vi "Generate Simulated Channel Block.vi"(8 "error in (no error)":errorcluster, 9 "Target Size (bytes)":i32, 10 "Number of Channels":i32, 11 "Simulated VeriStand Engine in":refnum<class "Simulated VeriStand Engine.lvclass">) -> (0 "error out":errorcluster, 1 "Actual Size (bytes)":i32, 2 "Channels":T1[](array[typedef]), 3 "Simulated VeriStand Engine out":refnum<class "Simulated VeriStand Engine.lvclass">)   [LabVIEW 2016, in "Simulated VeriStand Engine.lvclass"]
uses:
  Simulated VeriStand Engine.lvclass
  <vilib>/NI Veristand/VeriStand Data/Typedefs/Typedefs.Data Types.ctl
  <vilib>/NI Veristand/VeriStand Data/VeriStand Data.lvlib
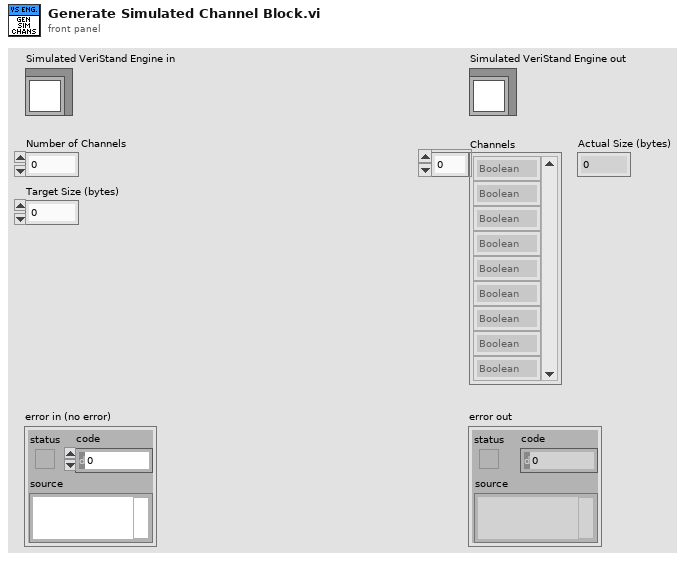
[diagram p1: front panel]
types:
  T1 = typedef "VeriStand Data.lvlib/Typedefs.Data Types.ctl" = enum16{"Boolean", "Single", "Double", "I8", "I16", "I32", "I64", "U8", "U16", "U32", "U64"}
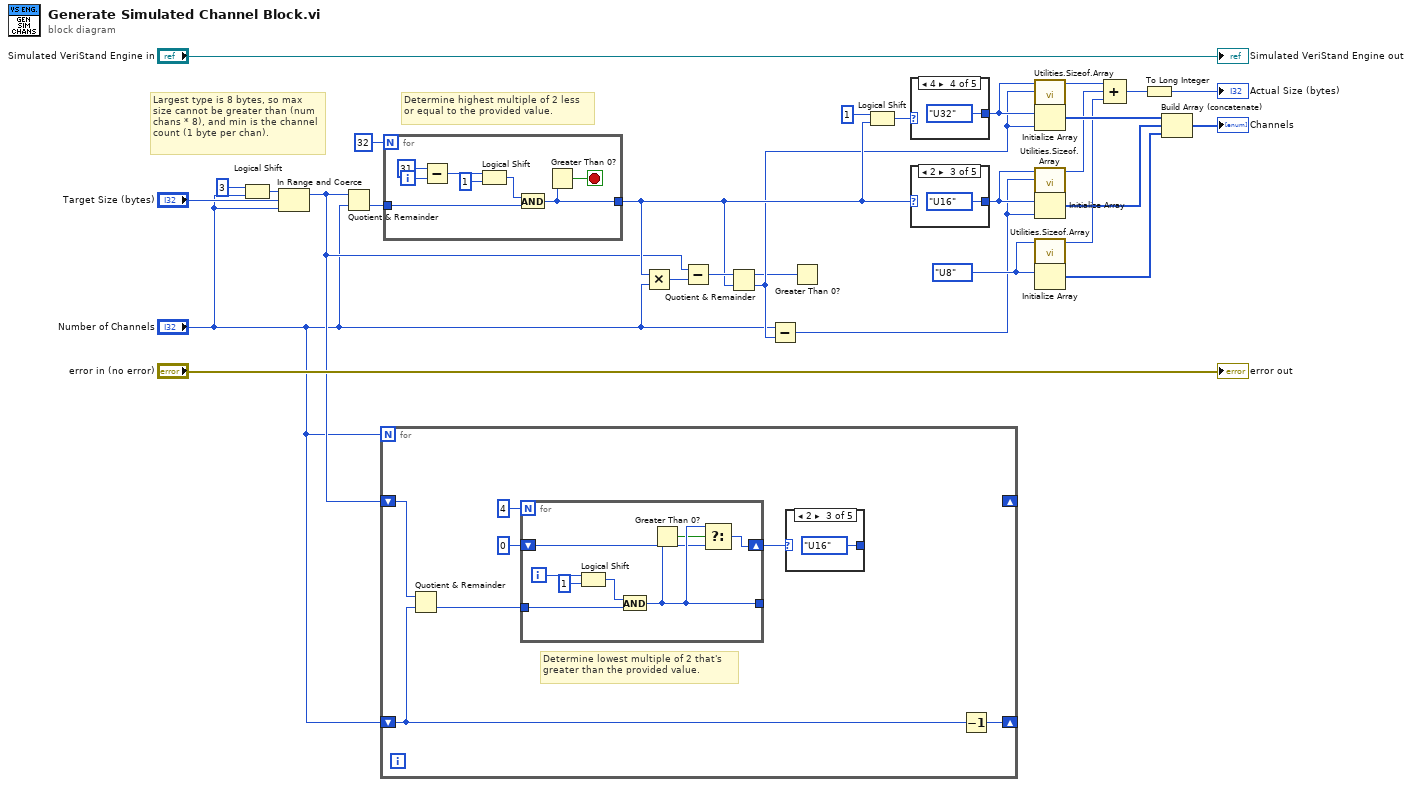
[diagram p0: block diagram]
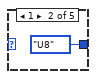
[diagram p3: hidden frame]
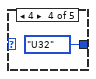
[diagram p4: hidden frame]
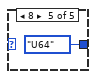
[diagram p5: hidden frame]
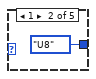
[diagram p7: hidden frame]
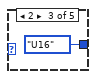
[diagram p8: hidden frame]
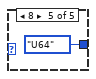
[diagram p9: hidden frame]
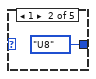
[diagram p11: hidden frame]
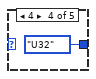
[diagram p12: hidden frame]
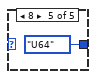
[diagram p13: hidden frame]
diagram:
  w16 = Typedefs.Data_Types."U8" ("data type")
  # "Determine highest multiple of 2 less or equal to the provided value."
  # "Largest type is 8 bytes, so max size cannot be greater than (num chans * 8), and min is the channel count (1 byte per chan)."
  n1 = Logical Shift(y=i16 3, x="Number of Channels") -> (x << y=w28:i32)
  n2 = In Range and Coerce(upper limit=w28, x="Target Size (bytes)", lower limit="Number of Channels") -> (coerced(x)=w2:i32)  [unwired: 1 out]
  n3 = Quotient & Remainder(x=w2, y="Number of Channels") -> (floor(x/y)=w27:i32)  [unwired: 1 out]
  n4 = for {
    N: "Number of Channels" -> [_]
    shift-right: _ -> [_]
    shift-left: w2 -> [w36]
    shift-right: [w37] -> _
    shift-left: "Number of Channels" -> [w35]
    # "Determine lowest multiple of 2 that's greater than the provided value."
    n5 = Quotient & Remainder(x=w36, y=w35) -> (floor(x/y)=w32:i32)  [unwired: 1 out]
    n6 = for {
      N: 4 -> [_]
      tunnel: w32 -> [w47]
      tunnel: [w45] -> _
      shift-right: [w44] -> w31
      shift-left: 0 ("x .and. y?") -> [w43]
      i -> [w46]
      n7 = Logical Shift(y=w46, x=1) -> (x << y=w48:i32)
      n8 = And(x=w48, y=w47) -> (x .and. y?=w45:i32)
      n9 = Greater Than 0?(x=w45) -> (x > 0?=w42:bool)
      n10 = Select(t=w45, s=w42, f=w43) -> (s? t:f=w44:i32)
    }
    n11 = case shown="2" w31 {
      tunnel: [_ Typedefs.Data_Types."U8" ("data type") Typedefs.Data_Types."U16" ("data type") Typedefs.Data_Types."U32" ("data type") Typedefs.Data_Types."U64" ("data type")] -> _
      frame 0, Default {
      }
      frame 1 {
      }
      frame 2 {
      }
      frame 4 {
      }
      frame 8 {
      }
    }
    n12 = Decrement(x=w35) -> (x-1=w37:i32)
  }
  n13 = for {
    N: 32 -> [_]
    tunnel: w27 -> [w53]
    tunnel: [w50] -> w7
    i -> [w52]
    stop <- w51 stop-if-true
    n14 = Subtract(x=31, y=w52) -> (x-y=w56:i32)
    n15 = Logical Shift(y=w56, x=1) -> (x << y=w54:i32)
    n16 = And(x=w54, y=w53) -> (x .and. y?=w50:i32)
    n17 = Greater Than 0?(x=w50) -> (x > 0?=w51:bool)
  }
  n18 = Multiply(x=w7, y="Number of Channels") -> (x*y=w25:i32)
  n19 = Subtract(x=w2, y=w25) -> (x-y=w8:i32)
  n20 = Quotient & Remainder(x=w8, y=w7) -> (x-y*floor(x/y)=w3:i32, floor(x/y)=w6:i32)
  n21 = Subtract(x="Number of Channels", y=w6) -> (x-y=w5:i32)
  n22 = Greater Than 0?(x=w3) -> ()  [unwired: 1 out]
  n23 = Logical Shift(y=i16 1, x=w7) -> (x << y=w23:i32)
  n24 = case shown="4" w23 {
    tunnel: [_ Typedefs.Data_Types."U8" ("data type") Typedefs.Data_Types."U16" ("data type") Typedefs.Data_Types."U32" ("data type") Typedefs.Data_Types."U64" ("data type")] -> w18
    frame 0, Default {
    }
    frame 1 {
    }
    frame 2 {
    }
    frame 4 {
    }
    frame 8 {
    }
  }
  n25 = case shown="2" w7 {
    tunnel: [_ Typedefs.Data_Types."U8" ("data type") Typedefs.Data_Types."U16" ("data type") Typedefs.Data_Types."U32" ("data type") Typedefs.Data_Types."U64" ("data type")] -> w17
    frame 0, Default {
    }
    frame 1 {
    }
    frame 2 {
    }
    frame 4 {
    }
    frame 8 {
    }
  }
  n26 = call <vilib>:"Utilities.Sizeof.Array.vi"("count"=w6, "data type"=w18) -> ("size"=w15:u64)  [unwired: 9 in]
  n27 = Initialize Array(w18, w6) -> (w22:T1[])
  n28 = call <vilib>:"Utilities.Sizeof.Array.vi"("count"=w5, "data type"=w17) -> ("size"=w14:u64)  [unwired: 9 in]
  n29 = Initialize Array(w17, w5) -> (w21:T1[])
  n30 = Initialize Array(w16) -> (w20:T1[], w4:i32)
  n31 = call <vilib>:"Utilities.Sizeof.Array.vi"("count"=w4, "data type"=w16) -> ("size"=w13:u64)  [unwired: 9 in]
  n32 = Compound Arithmetic op=ADD(w15, w14, w13) -> (w12:u64)
  n33 = To Long Integer(number=w12) -> (32bit integer=→"Actual Size (bytes)":i32)
  n34 = Build Array (concatenate)(w22, w21, w20) -> (→"Channels":T1[])
  "error out" <- "error in (no error)"
  "Simulated VeriStand Engine out" <- "Simulated VeriStand Engine in"
